vi "DashboardPush.vi"(5 "Joystick 0 Ref":T1, 7 "Joystick 1 Ref":T1) -> ()   [LabVIEW 2018]
uses:
  <vilib>/Rock Robotics/WPI/Joystick/WPI_JoystickDevRef.ctl
  <vilib>/Rock Robotics/WPI/Joystick/WPI_JoystickDeviceEnum.ctl
  e28dabe6-72c8-4d9b-bcee-39709893a3d3.vi
  6b09590c-8f19-4b7e-877c-f1124a14a17d.vi
  1cd4df9d-07b4-47b1-9361-2cbb9b342794.vi
  3ad63815-9e92-4927-9537-e4f1665bbc86.vi
  3818bb57-508c-4caa-99a3-3627e757767c.vi
  6295dfb8-7bb5-4d21-8815-7d68ced149fe.vi
  69aab131-d86d-4f55-ad43-4766d5f58e80.vi
  c3e94fa6-8c65-408c-b4b8-dd7b71f991a8.vi
  26d44c84-0892-4d1c-ad1a-86279a09e0cc.vi
  6918a5f6-b485-4e67-ab72-405280ef4693.vi
  11adc3a0-d4d2-454d-8758-117694ddcb4c.vi
  1a812ba0-d878-476d-99f2-b93886c55b51.vi
  4ab55bdd-9685-40f0-9085-ecc7bf01abd7.vi
  133b72f1-f6b5-40a0-849f-8c3469abb341.vi
  418ca814-9bf7-4181-a5ae-ea4e15d15a62.vi
  5b9a1c80-d2af-4722-947b-ad6779bb500a.vi
  bbae46cd-89b0-4a78-83b4-a5d1ddadd6d9.vi
  6394f793-1348-457d-85f4-7648f9013d39.vi
  47d326fc-03e5-451f-ae34-c9ea74063880.vi
  a9e42ba8-a108-4121-8da4-7ed463bc445a.vi
  e7382db6-2398-4bf7-9509-2739849d011a.vi
  fb3d1e40-1309-4105-9d60-3501161224b8.vi
  edb44874-fd78-454c-9bff-6d2a69ee6fec.vi
  dfb785ac-7a80-4692-ab1e-e9791fae54f3.vi
  5b13cb5e-6146-47d8-ae09-8b12801406e1.vi
  221b1552-0cc4-4389-bc13-d572fc4176ac.vi
  30f734cc-7591-4d07-939c-c5b43ee5df0c.vi
  d7311573-fb90-4913-8cda-848d1d3ce53b.vi
  7ba6df12-c395-4848-b3a1-04dcd1203c1b.vi
  6301e614-6b7f-47cf-b382-4b27c7e33111.vi
  d83519f1-9582-40c6-a23b-344b6b305b5b.vi
  6aad11fd-ae03-4511-b650-1fa0753debfc.vi
  3bc1cfba-3c18-4848-9658-0328ea52b25d.vi
  ee07aba5-9db9-42ab-a6d0-ff6a71bb383e.vi
  31b97e73-c245-4c28-83b2-b8b7bc5cac65.vi
  8687fe65-8d2d-4f02-ae89-6e8600396bf0.vi
  359c22e3-9c88-41c1-8194-a7f6db251ab3.vi
  9a35cad7-8924-4936-b892-f51ff88f3087.vi
  77a43352-c56d-4a82-a601-0e029bfbecdd.vi
  6c32de76-4603-4c98-9548-18c068db77e4.vi
  fb2c5630-2057-4e14-823f-31378c39dbf8.vi
  d6cbd67f-9b17-42bf-843e-f5ce2d93bab6.vi
  9a319e29-0bce-4b5a-a8ba-81b1ec785933.vi
  c84b3921-0e7b-4db5-8b5b-9ca439e6cec8.vi
  80ca6acc-a426-4631-8635-04e987b8dcbd.vi
  32f607b5-8f1a-4da3-a9f3-63ceddb82894.vi
  SensorReadings.vi
  RobotStates.vi
  Inputs_DriverStation.vi
  <vilib>/Rock Robotics/Network Tables/NT Write Number.vi
  <vilib>/Rock Robotics/Network Tables/NT Write Boolean.vi
  RefNums_DriverStation.vi
  <vilib>/Rock Robotics/Network Tables/NT Write String Array.vi
  Robot Global Data.vi
  <vilib>/Rock Robotics/Network Tables/NT Write String.vi
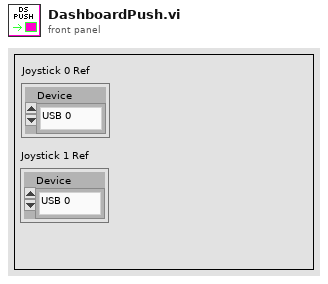
[diagram p1: front panel]
types:
  T1 = typedef "WPI_JoystickDevRef.ctl" = cluster{"Device":T2}
  T2 = typedef "WPI_JoystickDeviceEnum.ctl" = enum16{"USB 0", "USB 1", "USB 2", "USB 3", "USB 4", "USB 5"}
  T3 = cluster{"[0]":bool, "[1]":bool, "[2]":bool, "[3]":bool, "[4]":bool, "[5]":bool, "[6]":bool, "[7]":bool, "[8]":bool, "[9]":bool, "[10]":bool, "[11]":bool, "[12]":bool, "[13]":bool}
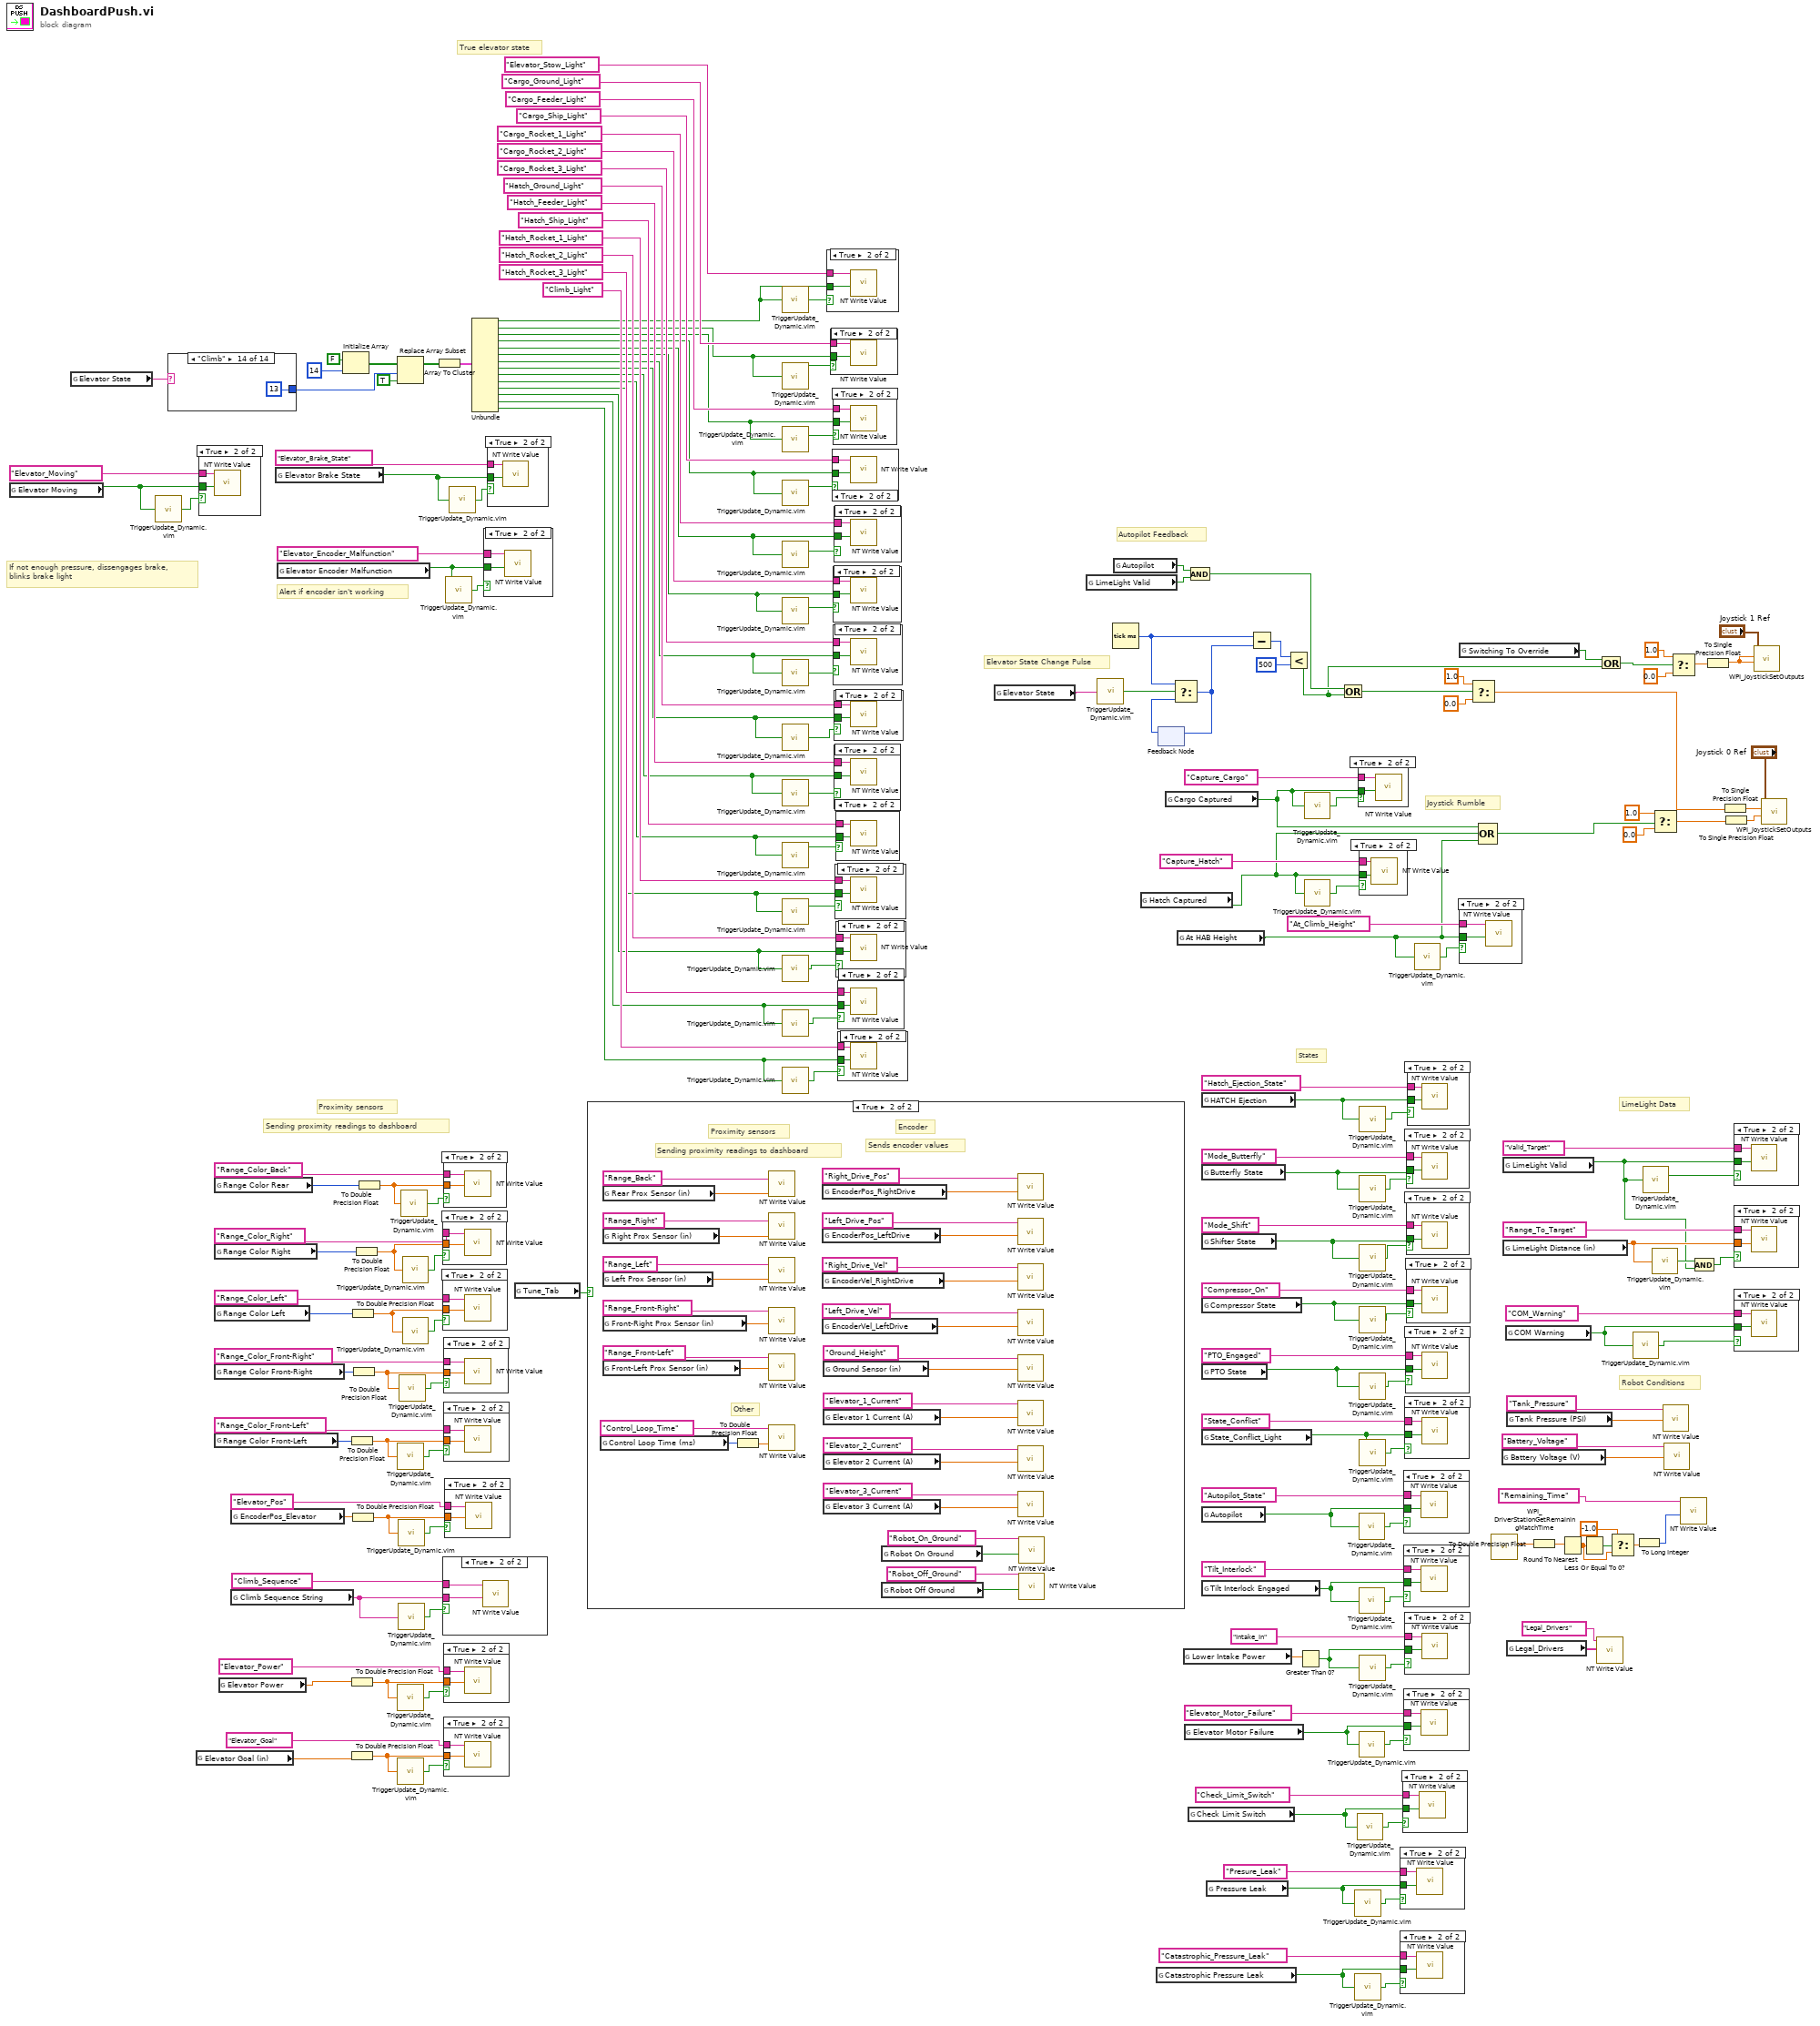
[diagram p0: block diagram]
diagram:
  # "Robot Conditions"
  # "States"
  # "Elevator State Change Pulse"
  # "LimeLight Data"
  # "Autopilot Feedback"
  # "Sending proximity readings to dashboard"
  # "Alert if encoder isn't working"
  # "If not enough pressure, dissengages brake,\nblinks brake light"
  # "Joystick Rumble"
  # "Proximity sensors"
  # "True elevator state"
  n1 = global read "RobotStates.vi" "Elevator Moving"() -> (w58:bool)
  n2 = global read "RobotStates.vi" "Elevator State"() -> (w164:string)
  n3 = call "TriggerUpdate_Dynamic.vim"("Trigger"=w58) -> ("Update"=w57:bool)
  n4 = case shown="\"Climb\"" w164 {
    tunnel: [0 1 2 3 4 5 6 7 8 9 10 11 12 13] -> w163
    frame "Elevator_Stow", Default {
    }
    frame "Cargo_Ground" {
    }
    frame "Cargo_Feeder" {
    }
    frame "Cargo_Ship" {
    }
    frame "Cargo_Rocket_1" {
    }
    frame "Cargo_Rocket_2" {
    }
    frame "Cargo_Rocket_3" {
    }
    frame "Hatch_Ground" {
    }
    frame "Hatch_Feeder" {
    }
    frame "Hatch_Ship" {
    }
    frame "Hatch_Rocket_1" {
    }
    frame "Hatch_Rocket_2" {
    }
    frame "Hatch_Rocket_3" {
    }
    frame "Climb" {
    }
  }
  n5 = global read "RobotStates.vi" "Elevator Goal (in)"() -> (w15:dbl)
  n6 = case shown="True" w57 {
    tunnel: "Elevator_Moving" ("Name") -> [_ w213]
    tunnel: w58 -> [_ w212]
    frame False {
    }
    frame True {
      n7 = call-poly <vilib>:"NT Write Value.vi"("Boolean"=w212, "Name"=w213) -> ()  [unwired: 9 in, 1 out]
    }
  }
  n8 = global read "SensorReadings.vi" "Range Color Rear"() -> (w190:u32)
  n9 = global read "SensorReadings.vi" "Range Color Right"() -> (w188:u32)
  n10 = global read "SensorReadings.vi" "Range Color Left"() -> (w186:u32)
  n11 = global read "SensorReadings.vi" "Range Color Front-Right"() -> (w184:u32)
  n12 = global read "SensorReadings.vi" "Range Color Front-Left"() -> (w159:u32)
  n13 = global read "RobotStates.vi" "Elevator Power"() -> (w19:dbl)
  n14 = global read "SensorReadings.vi" "EncoderPos_Elevator"() -> (w38:dbl)
  n15 = global read "RobotStates.vi" "Climb Sequence String"() -> (w35:string)
  n16 = global read "RobotStates.vi" "Elevator Brake State"() -> (w99:bool)
  n17 = global read "SensorReadings.vi" "Elevator Encoder Malfunction"() -> (w53:bool)
  n18 = Initialize Array(FALSE, 14 ("dimension size")) -> (w169:bool[])
  n19 = To Double Precision Float(number=w159) -> (double precision float=w103:dbl)
  n20 = To Double Precision Float(number=w19) -> (double precision float=w22:dbl)
  n21 = To Double Precision Float(number=w15) -> (double precision float=w18:dbl)
  n22 = To Double Precision Float(number=w186) -> (double precision float=w107:dbl)
  n23 = To Double Precision Float(number=w38) -> (double precision float=w41:dbl)
  n24 = To Double Precision Float(number=w184) -> (double precision float=w105:dbl)
  n25 = To Double Precision Float(number=w188) -> (double precision float=w109:dbl)
  n26 = To Double Precision Float(number=w190) -> (double precision float=w111:dbl)
  n27 = Replace Array Subset(array=w169, new element=TRUE ("new element/subarray"), index=w163) -> (w167:bool[])
  n28 = call "TriggerUpdate_Dynamic.vim"("Trigger"=w103) -> ("Update"=w102:bool)
  n29 = call "TriggerUpdate_Dynamic.vim"("Trigger"=w22) -> ("Update"=w21:bool)
  n30 = call "TriggerUpdate_Dynamic.vim"("Trigger"=w18) -> ("Update"=w17:bool)
  n31 = call "TriggerUpdate_Dynamic.vim"("Trigger"=w41) -> ("Update"=w40:bool)
  n32 = call "TriggerUpdate_Dynamic.vim"("Trigger"=w35) -> ("Update"=w37:bool)
  n33 = call "TriggerUpdate_Dynamic.vim"("Trigger"=w105) -> ("Update"=w104:bool)
  n34 = call "TriggerUpdate_Dynamic.vim"("Trigger"=w111) -> ("Update"=w110:bool)
  n35 = call "TriggerUpdate_Dynamic.vim"("Trigger"=w109) -> ("Update"=w108:bool)
  n36 = call "TriggerUpdate_Dynamic.vim"("Trigger"=w107) -> ("Update"=w106:bool)
  n37 = Array To Cluster(array=w167) -> (cluster=w166:T3)
  n38 = case shown="True" w108 {
    tunnel: "Range_Color_Right" ("refnum name") -> [_ w215]
    tunnel: w109 -> [_ w214]
    frame False {
    }
    frame True {
      n39 = call-poly <vilib>:"NT Write Value.vi"("Numeric"=w214, "Name"=w215) -> ()  [unwired: 9 in, 1 out]
    }
  }
  n40 = case shown="True" w106 {
    tunnel: "Range_Color_Left" ("refnum name") -> [_ w217]
    tunnel: w107 -> [_ w216]
    frame False {
    }
    frame True {
      n41 = call-poly <vilib>:"NT Write Value.vi"("Numeric"=w216, "Name"=w217) -> ()  [unwired: 9 in, 1 out]
    }
  }
  n42 = case shown="True" w37 {
    tunnel: "Climb_Sequence" ("Name") -> [_ w219]
    tunnel: w35 -> [_ w218]
    frame False {
    }
    frame True {
      n43 = call-poly <vilib>:"NT Write Value.vi"("String"=w218, "Name"=w219) -> ()  [unwired: 9 in, 1 out]
    }
  }
  n44 = case shown="True" w110 {
    tunnel: "Range_Color_Back" ("refnum name") -> [_ w221]
    tunnel: w111 -> [_ w220]
    frame False {
    }
    frame True {
      n45 = call-poly <vilib>:"NT Write Value.vi"("Numeric"=w220, "Name"=w221) -> ()  [unwired: 9 in, 1 out]
    }
  }
  n46 = case shown="True" w104 {
    tunnel: "Range_Color_Front-Right" ("refnum name") -> [_ w223]
    tunnel: w105 -> [_ w222]
    frame False {
    }
    frame True {
      n47 = call-poly <vilib>:"NT Write Value.vi"("Numeric"=w222, "Name"=w223) -> ()  [unwired: 9 in, 1 out]
    }
  }
  n48 = case shown="True" w102 {
    tunnel: w103 -> [_ w225]
    tunnel: "Range_Color_Front-Left" ("refnum name") -> [_ w224]
    frame False {
    }
    frame True {
      n49 = call-poly <vilib>:"NT Write Value.vi"("Numeric"=w225, "Name"=w224) -> ()  [unwired: 9 in, 1 out]
    }
  }
  n50 = case shown="True" w21 {
    tunnel: w22 -> [_ w227]
    tunnel: "Elevator_Power" ("Name") -> [_ w226]
    frame False {
    }
    frame True {
      n51 = call-poly <vilib>:"NT Write Value.vi"("Numeric"=w227, "Name"=w226) -> ()  [unwired: 9 in, 1 out]
    }
  }
  n52 = case shown="True" w17 {
    tunnel: w18 -> [_ w229]
    tunnel: "Elevator_Goal" ("Name") -> [_ w228]
    frame False {
    }
    frame True {
      n53 = call-poly <vilib>:"NT Write Value.vi"("Numeric"=w229, "Name"=w228) -> ()  [unwired: 9 in, 1 out]
    }
  }
  n54 = case shown="True" w40 {
    tunnel: w41 -> [_ w231]
    tunnel: "Elevator_Pos" ("Name") -> [_ w230]
    frame False {
    }
    frame True {
      n55 = call-poly <vilib>:"NT Write Value.vi"("Numeric"=w231, "Name"=w230) -> ()  [unwired: 9 in, 1 out]
    }
  }
  n56 = call "TriggerUpdate_Dynamic.vim"("Trigger"=w53) -> ("Update"=w100:bool)
  n57 = call "TriggerUpdate_Dynamic.vim"("Trigger"=w99) -> ("Update"=w98:bool)
  n58 = Unbundle(w166) -> ("[0]"=w154:bool, "[1]"=w152:bool, "[2]"=w150:bool, "[3]"=w148:bool, "[4]"=w146:bool, "[5]"=w144:bool, "[6]"=w142:bool, "[7]"=w140:bool, "[8]"=w138:bool, "[9]"=w136:bool, "[10]"=w134:bool, "[11]"=w132:bool, "[12]"=w130:bool, "[13]"=w128:bool)
  n59 = case shown="True" w100 {
    tunnel: "Elevator_Encoder_Malfunction" ("Name") -> [_ w233]
    tunnel: w53 -> [_ w232]
    frame False {
    }
    frame True {
      n60 = call-poly <vilib>:"NT Write Value.vi"("Boolean"=w232, "Name"=w233) -> ()  [unwired: 9 in, 1 out]
    }
  }
  n61 = case shown="True" w98 {
    tunnel: "Elevator_Brake_State" ("Name") -> [_ w235]
    tunnel: w99 -> [_ w234]
    frame False {
    }
    frame True {
      n62 = call-poly <vilib>:"NT Write Value.vi"("Boolean"=w234, "Name"=w235) -> ()  [unwired: 9 in, 1 out]
    }
  }
  n63 = global read "Inputs_DriverStation.vi" "Tune_Tab"() -> (w101:bool)
  n64 = case shown="True" w101 {
    frame False {
    }
    frame True {
      # "Sending proximity readings to dashboard"
      # "Proximity sensors"
      # "Sends encoder values"
      # "Other"
      # "Encoder"
      n65 = global read "SensorReadings.vi" "Control Loop Time (ms)"() -> (w249:u32)
      n66 = global read "SensorReadings.vi" "Rear Prox Sensor (in)"() -> (w267:dbl)
      n67 = global read "SensorReadings.vi" "Right Prox Sensor (in)"() -> (w265:dbl)
      n68 = global read "SensorReadings.vi" "Left Prox Sensor (in)"() -> (w263:dbl)
      n69 = global read "SensorReadings.vi" "Front-Right Prox Sensor (in)"() -> (w261:dbl)
      n70 = global read "SensorReadings.vi" "Front-Left Prox Sensor (in)"() -> (w251:dbl)
      n71 = To Double Precision Float(number=w249) -> (double precision float=w248:dbl)
      n72 = call-poly <vilib>:"NT Write Value.vi"("Numeric"=w267, "Name"="Range_Back") -> ()  [unwired: 9 in, 1 out]
      n73 = call-poly <vilib>:"NT Write Value.vi"("Numeric"=w265, "Name"="Range_Right") -> ()  [unwired: 9 in, 1 out]
      n74 = call-poly <vilib>:"NT Write Value.vi"("Numeric"=w263, "Name"="Range_Left") -> ()  [unwired: 9 in, 1 out]
      n75 = call-poly <vilib>:"NT Write Value.vi"("Numeric"=w261, "Name"="Range_Front-Right") -> ()  [unwired: 9 in, 1 out]
      n76 = call-poly <vilib>:"NT Write Value.vi"("Numeric"=w251, "Name"="Range_Front-Left") -> ()  [unwired: 9 in, 1 out]
      n77 = call-poly <vilib>:"NT Write Value.vi"("Numeric"=w248, "Name"="Control_Loop_Time") -> ()  [unwired: 9 in, 1 out]
      n78 = global read "SensorReadings.vi" "EncoderPos_RightDrive"() -> (w260:dbl)
      n79 = global read "SensorReadings.vi" "EncoderPos_LeftDrive"() -> (w258:dbl)
      n80 = global read "SensorReadings.vi" "EncoderVel_RightDrive"() -> (w256:dbl)
      n81 = global read "SensorReadings.vi" "EncoderVel_LeftDrive"() -> (w254:dbl)
      n82 = global read "SensorReadings.vi" "Ground Sensor (in)"() -> (w246:dbl)
      n83 = global read "SensorReadings.vi" "Elevator 1 Current (A)"() -> (w244:dbl)
      n84 = global read "SensorReadings.vi" "Elevator 2 Current (A)"() -> (w242:dbl)
      n85 = global read "SensorReadings.vi" "Elevator 3 Current (A)"() -> (w240:dbl)
      n86 = global read "SensorReadings.vi" "Robot On Ground"() -> (w238:bool)
      n87 = global read "SensorReadings.vi" "Robot Off Ground"() -> (w239:bool)
      n88 = call-poly <vilib>:"NT Write Value.vi"("Numeric"=w260, "Name"="Right_Drive_Pos") -> ()  [unwired: 9 in, 1 out]
      n89 = call-poly <vilib>:"NT Write Value.vi"("Numeric"=w258, "Name"="Left_Drive_Pos") -> ()  [unwired: 9 in, 1 out]
      n90 = call-poly <vilib>:"NT Write Value.vi"("Numeric"=w256, "Name"="Right_Drive_Vel") -> ()  [unwired: 9 in, 1 out]
      n91 = call-poly <vilib>:"NT Write Value.vi"("Numeric"=w254, "Name"="Left_Drive_Vel") -> ()  [unwired: 9 in, 1 out]
      n92 = call-poly <vilib>:"NT Write Value.vi"("Numeric"=w246, "Name"="Ground_Height") -> ()  [unwired: 9 in, 1 out]
      n93 = call-poly <vilib>:"NT Write Value.vi"("Numeric"=w244, "Name"="Elevator_1_Current") -> ()  [unwired: 9 in, 1 out]
      n94 = call-poly <vilib>:"NT Write Value.vi"("Numeric"=w242, "Name"="Elevator_2_Current") -> ()  [unwired: 9 in, 1 out]
      n95 = call-poly <vilib>:"NT Write Value.vi"("Numeric"=w240, "Name"="Elevator_3_Current") -> ()  [unwired: 9 in, 1 out]
      n96 = call-poly <vilib>:"NT Write Value.vi"("Boolean"=w238, "Name"="Robot_On_Ground") -> ()  [unwired: 9 in, 1 out]
      n97 = call-poly <vilib>:"NT Write Value.vi"("Boolean"=w239, "Name"="Robot_Off_Ground") -> ()  [unwired: 9 in, 1 out]
    }
  }
  n98 = call "TriggerUpdate_Dynamic.vim"("Trigger"=w154) -> ("Update"=w153:bool)
  n99 = call "TriggerUpdate_Dynamic.vim"("Trigger"=w152) -> ("Update"=w151:bool)
  n100 = call "TriggerUpdate_Dynamic.vim"("Trigger"=w150) -> ("Update"=w149:bool)
  n101 = call "TriggerUpdate_Dynamic.vim"("Trigger"=w148) -> ("Update"=w147:bool)
  n102 = call "TriggerUpdate_Dynamic.vim"("Trigger"=w146) -> ("Update"=w145:bool)
  n103 = call "TriggerUpdate_Dynamic.vim"("Trigger"=w144) -> ("Update"=w143:bool)
  n104 = call "TriggerUpdate_Dynamic.vim"("Trigger"=w142) -> ("Update"=w141:bool)
  n105 = call "TriggerUpdate_Dynamic.vim"("Trigger"=w140) -> ("Update"=w139:bool)
  n106 = call "TriggerUpdate_Dynamic.vim"("Trigger"=w138) -> ("Update"=w137:bool)
  n107 = call "TriggerUpdate_Dynamic.vim"("Trigger"=w136) -> ("Update"=w135:bool)
  n108 = call "TriggerUpdate_Dynamic.vim"("Trigger"=w134) -> ("Update"=w133:bool)
  n109 = call "TriggerUpdate_Dynamic.vim"("Trigger"=w132) -> ("Update"=w131:bool)
  n110 = call "TriggerUpdate_Dynamic.vim"("Trigger"=w130) -> ("Update"=w129:bool)
  n111 = call "TriggerUpdate_Dynamic.vim"("Trigger"=w128) -> ("Update"=w127:bool)
  n112 = case shown="True" w153 {
    tunnel: "Elevator_Stow_Light" ("refnum name") -> [_ w270]
    tunnel: w154 -> [_ w269]
    frame False {
    }
    frame True {
      n113 = call-poly <vilib>:"NT Write Value.vi"("Boolean"=w269, "Name"=w270) -> ()  [unwired: 9 in, 1 out]
    }
  }
  n114 = case shown="True" w151 {
    tunnel: "Cargo_Ground_Light" ("refnum name") -> [_ w272]
    tunnel: w152 -> [_ w271]
    frame False {
    }
    frame True {
      n115 = call-poly <vilib>:"NT Write Value.vi"("Boolean"=w271, "Name"=w272) -> ()  [unwired: 9 in, 1 out]
    }
  }
  n116 = case shown="True" w147 {
    tunnel: "Cargo_Ship_Light" ("refnum name") -> [_ w274]
    tunnel: w148 -> [_ w273]
    frame False {
    }
    frame True {
      n117 = call-poly <vilib>:"NT Write Value.vi"("Boolean"=w273, "Name"=w274) -> ()  [unwired: 9 in, 1 out]
    }
  }
  n118 = case shown="True" w149 {
    tunnel: "Cargo_Feeder_Light" ("refnum name") -> [_ w276]
    tunnel: w150 -> [_ w275]
    frame False {
    }
    frame True {
      n119 = call-poly <vilib>:"NT Write Value.vi"("Boolean"=w275, "Name"=w276) -> ()  [unwired: 9 in, 1 out]
    }
  }
  n120 = case shown="True" w143 {
    tunnel: "Cargo_Rocket_2_Light" ("refnum name") -> [_ w278]
    tunnel: w144 -> [_ w277]
    frame False {
    }
    frame True {
      n121 = call-poly <vilib>:"NT Write Value.vi"("Boolean"=w277, "Name"=w278) -> ()  [unwired: 9 in, 1 out]
    }
  }
  n122 = case shown="True" w141 {
    tunnel: "Cargo_Rocket_3_Light" ("refnum name") -> [_ w280]
    tunnel: w142 -> [_ w279]
    frame False {
    }
    frame True {
      n123 = call-poly <vilib>:"NT Write Value.vi"("Boolean"=w279, "Name"=w280) -> ()  [unwired: 9 in, 1 out]
    }
  }
  n124 = case shown="True" w145 {
    tunnel: "Cargo_Rocket_1_Light" ("refnum name") -> [_ w282]
    tunnel: w146 -> [_ w281]
    frame False {
    }
    frame True {
      n125 = call-poly <vilib>:"NT Write Value.vi"("Boolean"=w281, "Name"=w282) -> ()  [unwired: 9 in, 1 out]
    }
  }
  n126 = case shown="True" w139 {
    tunnel: "Hatch_Ground_Light" ("refnum name") -> [_ w284]
    tunnel: w140 -> [_ w283]
    frame False {
    }
    frame True {
      n127 = call-poly <vilib>:"NT Write Value.vi"("Boolean"=w283, "Name"=w284) -> ()  [unwired: 9 in, 1 out]
    }
  }
  n128 = case shown="True" w137 {
    tunnel: "Hatch_Feeder_Light" ("refnum name") -> [_ w286]
    tunnel: w138 -> [_ w285]
    frame False {
    }
    frame True {
      n129 = call-poly <vilib>:"NT Write Value.vi"("Boolean"=w285, "Name"=w286) -> ()  [unwired: 9 in, 1 out]
    }
  }
  n130 = case shown="True" w133 {
    tunnel: "Hatch_Rocket_1_Light" ("refnum name") -> [_ w288]
    tunnel: w134 -> [_ w287]
    frame False {
    }
    frame True {
      n131 = call-poly <vilib>:"NT Write Value.vi"("Boolean"=w287, "Name"=w288) -> ()  [unwired: 9 in, 1 out]
    }
  }
  n132 = case shown="True" w135 {
    tunnel: "Hatch_Ship_Light" ("refnum name") -> [_ w290]
    tunnel: w136 -> [_ w289]
    frame False {
    }
    frame True {
      n133 = call-poly <vilib>:"NT Write Value.vi"("Boolean"=w289, "Name"=w290) -> ()  [unwired: 9 in, 1 out]
    }
  }
  n134 = case shown="True" w131 {
    tunnel: "Hatch_Rocket_2_Light" ("refnum name") -> [_ w292]
    tunnel: w132 -> [_ w291]
    frame False {
    }
    frame True {
      n135 = call-poly <vilib>:"NT Write Value.vi"("Boolean"=w291, "Name"=w292) -> ()  [unwired: 9 in, 1 out]
    }
  }
  n136 = case shown="True" w129 {
    tunnel: "Hatch_Rocket_3_Light" ("refnum name") -> [_ w294]
    tunnel: w130 -> [_ w293]
    frame False {
    }
    frame True {
      n137 = call-poly <vilib>:"NT Write Value.vi"("Boolean"=w293, "Name"=w294) -> ()  [unwired: 9 in, 1 out]
    }
  }
  n138 = case shown="True" w127 {
    tunnel: "Climb_Light" ("refnum name") -> [_ w296]
    tunnel: w128 -> [_ w295]
    frame False {
    }
    frame True {
      n139 = call-poly <vilib>:"NT Write Value.vi"("Boolean"=w295, "Name"=w296) -> ()  [unwired: 9 in, 1 out]
    }
  }
  n140 = global read "RobotStates.vi" "Elevator State"() -> (w73:string)
  n141 = global read "SensorReadings.vi" "LimeLight Valid"() -> (w96:bool)
  n142 = call "TriggerUpdate_Dynamic.vim"("Trigger"=w73) -> ("Update"=w65:bool)
  n143 = Tick Count (ms)() -> (millisecond timer value=w69:u32)
  n144 = global read "RobotStates.vi" "Autopilot"() -> (w97:bool)
  n145 = global read "SensorReadings.vi" "Hatch Captured"() -> (w74:bool)
  n146 = global read "SensorReadings.vi" "Catastrophic Pressure Leak"() -> (w1:bool)
  n147 = feedback #1() -> (w70:u32)  [unwired: 1 in]
  n148 = global read "SensorReadings.vi" "Cargo Captured"() -> (w125:bool)
  n149 = Select(t=w69, s=w65, f=w70) -> (s? t:f=w68:u32)
  n150 = feedback-in #1(w68) -> ()
  n151 = global read "SensorReadings.vi" "At HAB Height"() -> (w42:bool)
  n152 = global read "RobotStates.vi" "Lower Intake Power"() -> (w32:dbl)
  n153 = global read "RobotStates.vi" "Elevator Motor Failure"() -> (w12:bool)
  n154 = And(x=w97, y=w96) -> (x .and. y?=w72:bool)
  n155 = global read "RobotStates.vi" "Check Limit Switch"() -> (w9:bool)
  n156 = global read "RobotStates.vi" "HATCH Ejection"() -> (w123:bool)
  n157 = global read "RobotStates.vi" "Butterfly State"() -> (w121:bool)
  n158 = global read "RobotStates.vi" "Shifter State"() -> (w119:bool)
  n159 = global read "RobotStates.vi" "Compressor State"() -> (w117:bool)
  n160 = global read "RobotStates.vi" "PTO State"() -> (w115:bool)
  n161 = global read "RobotStates.vi" "State_Conflict_Light"() -> (w113:bool)
  n162 = global read "RobotStates.vi" "Autopilot"() -> (w85:bool)
  n163 = global read "RobotStates.vi" "Tilt Interlock Engaged"() -> (w49:bool)
  n164 = global read "SensorReadings.vi" "Pressure Leak"() -> (w2:bool)
  n165 = Subtract(x=w69, y=w68) -> (x-y=w67:u32)
  n166 = Less?(x=w67, y=u32 500) -> (x < y?=w47:bool)
  n167 = Greater Than 0?(x=w32) -> (x > 0?=w31:bool)
  n168 = call "TriggerUpdate_Dynamic.vim"("Trigger"=w125) -> ("Update"=w124:bool)
  n169 = call "TriggerUpdate_Dynamic.vim"("Trigger"=w74) -> ("Update"=w126:bool)
  n170 = Or(x=w72, y=w47) -> (x .or. y?=w71:bool)
  n171 = call "TriggerUpdate_Dynamic.vim"("Trigger"=w2) -> ("Update"=w5:bool)
  n172 = call "TriggerUpdate_Dynamic.vim"("Trigger"=w1) -> ("Update"=w3:bool)
  n173 = call "TriggerUpdate_Dynamic.vim"("Trigger"=w9) -> ("Update"=w10:bool)
  n174 = case shown="True" w124 {
    tunnel: "Capture_Cargo" ("Name") -> [_ w298]
    tunnel: w125 -> [_ w297]
    frame False {
    }
    frame True {
      n175 = call-poly <vilib>:"NT Write Value.vi"("Boolean"=w297, "Name"=w298) -> ()  [unwired: 9 in, 1 out]
    }
  }
  n176 = call "TriggerUpdate_Dynamic.vim"("Trigger"=w85) -> ("Update"=w84:bool)
  n177 = call "TriggerUpdate_Dynamic.vim"("Trigger"=w49) -> ("Update"=w48:bool)
  n178 = call "TriggerUpdate_Dynamic.vim"("Trigger"=w12) -> ("Update"=w13:bool)
  n179 = case shown="True" w126 {
    tunnel: "Capture_Hatch" ("Name") -> [_ w300]
    tunnel: w74 -> [_ w299]
    frame False {
    }
    frame True {
      n180 = call-poly <vilib>:"NT Write Value.vi"("Boolean"=w299, "Name"=w300) -> ()  [unwired: 9 in, 1 out]
    }
  }
  n181 = call "TriggerUpdate_Dynamic.vim"("Trigger"=w123) -> ("Update"=w122:bool)
  n182 = call "TriggerUpdate_Dynamic.vim"("Trigger"=w121) -> ("Update"=w120:bool)
  n183 = call "TriggerUpdate_Dynamic.vim"("Trigger"=w119) -> ("Update"=w118:bool)
  n184 = call "TriggerUpdate_Dynamic.vim"("Trigger"=w117) -> ("Update"=w116:bool)
  n185 = call "TriggerUpdate_Dynamic.vim"("Trigger"=w115) -> ("Update"=w114:bool)
  n186 = call "TriggerUpdate_Dynamic.vim"("Trigger"=w113) -> ("Update"=w112:bool)
  n187 = call "TriggerUpdate_Dynamic.vim"("Trigger"=w31) -> ("Update"=w33:bool)
  n188 = case shown="True" w5 {
    tunnel: w2 -> [_ w302]
    tunnel: "Presure_Leak" ("Name") -> [_ w301]
    frame False {
    }
    frame True {
      n189 = call-poly <vilib>:"NT Write Value.vi"("Boolean"=w302, "Name"=w301) -> ()  [unwired: 9 in, 1 out]
    }
  }
  n190 = case shown="True" w3 {
    tunnel: w1 -> [_ w304]
    tunnel: "Catastrophic_Pressure_Leak" ("Name") -> [_ w303]
    frame False {
    }
    frame True {
      n191 = call-poly <vilib>:"NT Write Value.vi"("Boolean"=w304, "Name"=w303) -> ()  [unwired: 9 in, 1 out]
    }
  }
  n192 = case shown="True" w10 {
    tunnel: w9 -> [_ w306]
    tunnel: "Check_Limit_Switch" ("Name") -> [_ w305]
    frame False {
    }
    frame True {
      n193 = call-poly <vilib>:"NT Write Value.vi"("Boolean"=w306, "Name"=w305) -> ()  [unwired: 9 in, 1 out]
    }
  }
  n194 = case shown="True" w84 {
    tunnel: w85 -> [_ w308]
    tunnel: "Autopilot_State" ("Name") -> [_ w307]
    frame False {
    }
    frame True {
      n195 = call-poly <vilib>:"NT Write Value.vi"("Boolean"=w308, "Name"=w307) -> ()  [unwired: 9 in, 1 out]
    }
  }
  n196 = case shown="True" w48 {
    tunnel: w49 -> [_ w310]
    tunnel: "Tilt_Interlock" ("Name") -> [_ w309]
    frame False {
    }
    frame True {
      n197 = call-poly <vilib>:"NT Write Value.vi"("Boolean"=w310, "Name"=w309) -> ()  [unwired: 9 in, 1 out]
    }
  }
  n198 = case shown="True" w13 {
    tunnel: w12 -> [_ w312]
    tunnel: "Elevator_Motor_Failure" ("Name") -> [_ w311]
    frame False {
    }
    frame True {
      n199 = call-poly <vilib>:"NT Write Value.vi"("Boolean"=w312, "Name"=w311) -> ()  [unwired: 9 in, 1 out]
    }
  }
  n200 = case shown="True" w112 {
    tunnel: w113 -> [_ w314]
    tunnel: "State_Conflict" ("Name") -> [_ w313]
    frame False {
    }
    frame True {
      n201 = call-poly <vilib>:"NT Write Value.vi"("Boolean"=w314, "Name"=w313) -> ()  [unwired: 9 in, 1 out]
    }
  }
  n202 = case shown="True" w33 {
    tunnel: w31 -> [_ w316]
    tunnel: "Intake_In" ("Name") -> [_ w315]
    frame False {
    }
    frame True {
      n203 = call-poly <vilib>:"NT Write Value.vi"("Boolean"=w316, "Name"=w315) -> ()  [unwired: 9 in, 1 out]
    }
  }
  n204 = case shown="True" w114 {
    tunnel: "PTO_Engaged" ("Name") -> [_ w318]
    tunnel: w115 -> [_ w317]
    frame False {
    }
    frame True {
      n205 = call-poly <vilib>:"NT Write Value.vi"("Boolean"=w317, "Name"=w318) -> ()  [unwired: 9 in, 1 out]
    }
  }
  n206 = case shown="True" w120 {
    tunnel: "Mode_Butterfly" ("Name") -> [_ w320]
    tunnel: w121 -> [_ w319]
    frame False {
    }
    frame True {
      n207 = call-poly <vilib>:"NT Write Value.vi"("Boolean"=w319, "Name"=w320) -> ()  [unwired: 9 in, 1 out]
    }
  }
  n208 = case shown="True" w118 {
    tunnel: "Mode_Shift" ("Name") -> [_ w322]
    tunnel: w119 -> [_ w321]
    frame False {
    }
    frame True {
      n209 = call-poly <vilib>:"NT Write Value.vi"("Boolean"=w321, "Name"=w322) -> ()  [unwired: 9 in, 1 out]
    }
  }
  n210 = case shown="True" w116 {
    tunnel: "Compressor_On" ("Name") -> [_ w324]
    tunnel: w117 -> [_ w323]
    frame False {
    }
    frame True {
      n211 = call-poly <vilib>:"NT Write Value.vi"("Boolean"=w323, "Name"=w324) -> ()  [unwired: 9 in, 1 out]
    }
  }
  n212 = case shown="True" w122 {
    tunnel: "Hatch_Ejection_State" ("Name") -> [_ w326]
    tunnel: w123 -> [_ w325]
    frame False {
    }
    frame True {
      n213 = call-poly <vilib>:"NT Write Value.vi"("Boolean"=w325, "Name"=w326) -> ()  [unwired: 9 in, 1 out]
    }
  }
  n214 = call "TriggerUpdate_Dynamic.vim"("Trigger"=w42) -> ("Update"=w43:bool)
  n215 = global read "Inputs_DriverStation.vi" "Switching To Override"() -> (w45:bool)
  n216 = case shown="True" w43 {
    tunnel: "At_Climb_Height" ("Name") -> [_ w328]
    tunnel: w42 -> [_ w327]
    frame False {
    }
    frame True {
      n217 = call-poly <vilib>:"NT Write Value.vi"("Boolean"=w327, "Name"=w328) -> ()  [unwired: 9 in, 1 out]
    }
  }
  n218 = Select(t=1.0, s=w71, f=0.0) -> (s? t:f=w89:dbl)
  n219 = Compound Arithmetic op=OR(w125, w74, w42) -> (w87:bool)
  n220 = call <vilib>:"WPI_DriverStationGetRemainingMatchTime.vi"() -> ("Match Time(s)"=w29:sgl)  [unwired: 10 in, 1 out]
  n221 = global read "SensorReadings.vi" "Battery Voltage (V)"() -> (w52:dbl)
  n222 = global read "SensorReadings.vi" "LimeLight Valid"() -> (w77:bool)
  n223 = global read "SensorReadings.vi" "LimeLight Distance (in)"() -> (w80:dbl)
  n224 = global read "RobotStates.vi" "COM Warning"() -> (w55:bool)
  n225 = global read "SensorReadings.vi" "Tank Pressure (PSI)"() -> (w76:dbl)
  n226 = global read "RefNums_DriverStation.vi" "Legal_Drivers"() -> (w8:string[])
  n227 = To Double Precision Float(number=w29) -> (double precision float=w28:dbl)
  n228 = Round To Nearest(number=w28) -> (nearest integer value=w26:dbl)
  n229 = Less Or Equal To 0?(x=w26) -> (x <= 0?=w27:bool)
  n230 = call-poly <vilib>:"NT Write Value.vi"("String Array"=w8, "Name"="Legal_Drivers") -> ()  [unwired: 9 in, 1 out]
  n231 = Or(x=w45, y=w47) -> (x .or. y?=w46:bool)
  n232 = Select(t=-1.0, s=w27, f=w26) -> (s? t:f=w25:dbl)
  n233 = call "TriggerUpdate_Dynamic.vim"("Trigger"=w55) -> ("Update"=w54:bool)
  n234 = To Long Integer(number=w25) -> (32bit integer=w24:i32)
  n235 = call "TriggerUpdate_Dynamic.vim"("Trigger"=w77) -> ("Update"=w82:bool)
  n236 = Select(t=1.0, s=w87, f=0.0) -> (s? t:f=w88:dbl)
  n237 = call "TriggerUpdate_Dynamic.vim"("Trigger"=w80) -> ("Update"=w79:bool)
  n238 = call-poly <vilib>:"NT Write Value.vi"("Numeric"=w76, "Name"="Tank_Pressure") -> ()  [unwired: 9 in, 1 out]
  n239 = call-poly <vilib>:"NT Write Value.vi"("Numeric"=w52, "Name"="Battery_Voltage") -> ()  [unwired: 9 in, 1 out]
  n240 = Select(t=1.0, s=w46, f=0.0) -> (s? t:f=w62:dbl)
  n241 = call-poly <vilib>:"NT Write Value.vi"("Numeric"=w24, "Name"="Remaining_Time") -> ()  [unwired: 9 in, 1 out]
  n242 = And(x=w79, y=w77) -> (x .and. y?=w78:bool)
  n243 = To Single Precision Float(number=w62) -> (single precision float=w60:sgl)
  n244 = To Single Precision Float(number=w89) -> (single precision float=w93:sgl)
  n245 = To Single Precision Float(number=w88) -> (single precision float=w90:sgl)
  n246 = case shown="True" w82 {
    tunnel: w77 -> [_ w330]
    tunnel: "Valid_Target" ("Name") -> [_ w329]
    frame False {
    }
    frame True {
      n247 = call-poly <vilib>:"NT Write Value.vi"("Boolean"=w330, "Name"=w329) -> ()  [unwired: 9 in, 1 out]
    }
  }
  n248 = case shown="True" w78 {
    tunnel: w80 -> [_ w332]
    tunnel: "Range_To_Target" ("Name") -> [_ w331]
    frame False {
    }
    frame True {
      n249 = call-poly <vilib>:"NT Write Value.vi"("Numeric"=w332, "Name"=w331) -> ()  [unwired: 9 in, 1 out]
    }
  }
  n250 = case shown="True" w54 {
    tunnel: w55 -> [_ w334]
    tunnel: "COM_Warning" ("Name") -> [_ w333]
    frame False {
    }
    frame True {
      n251 = call-poly <vilib>:"NT Write Value.vi"("Boolean"=w334, "Name"=w333) -> ()  [unwired: 9 in, 1 out]
    }
  }
  n252 = call <vilib>:"WPI_JoystickSetOutputs.vi"("Right Rumble"=w60, "Left Rumble"=w60, "JoystickDevRef"="Joystick 1 Ref") -> ()  [unwired: 7 in, 2 out]
  n253 = call <vilib>:"WPI_JoystickSetOutputs.vi"("Right Rumble"=w90, "Left Rumble"=w93, "JoystickDevRef"="Joystick 0 Ref") -> ()  [unwired: 7 in, 2 out]
